vi "tsa_Spectrum (AR).vi"(4 "method for sita^2":u16(ring) items=["Variance", "Energy"], 5 "onesided?":bool=TRUE, 6 "sampling frequency":dbl=1.0 format="%.2f", 7 "number of bins":i32=2000, 9 "noise":dbl[](array[numeric]) format="%.2f", 10 "sita^2":dbl, 11 "AR coefficients":dbl[](array[numeric])) -> (3 "PSD":cluster{"f0":dbl, "df":dbl, "Sx":dbl[]})   [LabVIEW 2014, in "NI_AALPro.lvlib"]
uses:
  NI_AALPro.lvlib
  NI_AALBase.lvlib
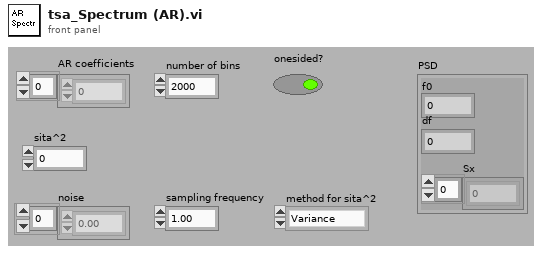
[diagram p1: front panel]
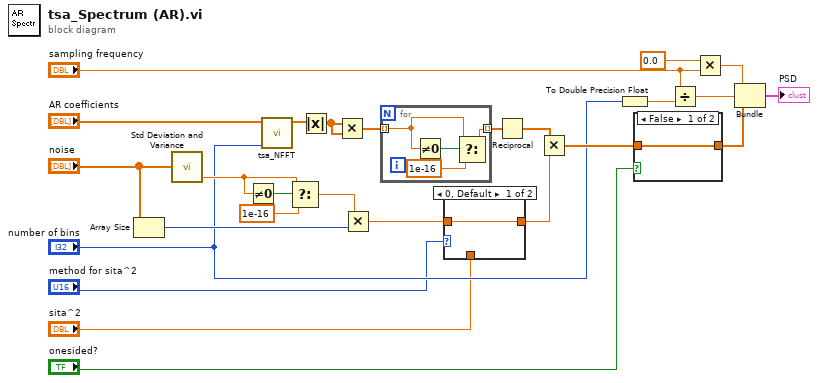
[diagram p0: block diagram]
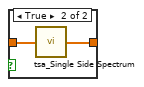
[diagram p2: hidden frame]
diagram:
  n1 = Array Size(array="noise") -> (size(s)=w15:i32)
  n2 = call "Std Deviation and Variance.vi"("X"="noise") -> ("variance"=w10:dbl)  [unwired: 1 in, 2 out]
  n3 = Not Equal To 0?(x=w10) -> (x != 0?=w13:bool)
  n4 = call "tsa_NFFT.vi"("nfft"="number of bins", "X"="AR coefficients") -> ("FFT {X}"=w19:cdb[])  [unwired: 8 in, 1 out]
  n5 = Select(t=w10, s=w13, f=1e-16) -> (s? t:f=w11:dbl)
  n6 = Absolute Value(x=w19) -> (abs(x)=w18:dbl[])
  n7 = Multiply(x=w18, y=w18) -> (x*y=w9:dbl[])
  n8 = Multiply(x=w11, y=w15) -> (x*y=w4:dbl)
  n9 = for {
    tunnel: w9 -> [w28] mode=indexing
    tunnel: [w27] -> w8 mode=indexing
    n10 = Not Equal To 0?(x=w28) -> (x != 0?=w30:bool)
    n11 = Select(t=w28, s=w30, f=1e-16) -> (s? t:f=w27:dbl)
  }
  n12 = case shown="0, Default" "method for sita^2" {
    tunnel: "sita^2" -> [_ w32]
    tunnel: w4 -> [w31 _]
    tunnel: [w31 w32] -> w3
    frame 0, Default {
    }
    frame 1 {
    }
  }
  n13 = Reciprocal(x=w8) -> (1/x=w17:dbl[])
  n14 = Multiply(x=w17, y=w3) -> (x*y=w14:dbl[])
  n15 = To Double Precision Float(number="number of bins") -> (double precision float=w21:dbl)
  n16 = case shown="False" "onesided?" {
    tunnel: [w33 w35] -> w16
    tunnel: w14 -> [w33 w34]
    frame False {
    }
    frame True {
      n17 = call "tsa_Single Side Spectrum.vi"("FFT {X}"=w34) -> ("FFT {X}"=w35:dbl[])
    }
  }
  n18 = Divide(x="sampling frequency", y=w21) -> (x/y=w25:dbl)
  n19 = Multiply(x=0.0 ("y"), y="sampling frequency") -> (x*y=w23:dbl)
  n20 = Bundle(w23, w25, "FFT {X}"=w16) -> (→"PSD":cluster{dbl, dbl, "FFT {X}":dbl[]})  [unwired: 1 in]
